vi "Compile 9759 RevB.vi"(8 "error in (no error)":errorcluster, 11 "Device Item Ref in":T2 format="%.0x") -> (0 "error out":errorcluster, 2 "9759 RevB":T1 {"Settings"."ControlCals"."ThetaLH (deg)" format="%.3f"; "Settings"."ControlCals"."ULHLag (sec)" format="%.3f"; "Settings"."ControlCals"."USLag (sec)" format="%.3f"; "Settings"."ControlCals"."TLead (sec)" format="%.3f"; "Settings"."ControlCals"."TLag (sec)" format="%.3f"}, 3 "Device Item Ref out":T2 format="%.0x")   [LabVIEW 2015, in "NI 9759 RevB Custom Device.lvlib"]
uses:
  NI 9759 RevB Custom Device.lvlib
  <vilib>/NI Veristand/Custom Device API/Custom Device Item Ref.ctl
  Shared/Types/9759 RevB.ctl
  Shared/9759 Constants and GUIDs.vi
  Shared/9759 Properties.vi
  <vilib>/NI VeriStand/Custom Device API/Custom Device API.lvlib
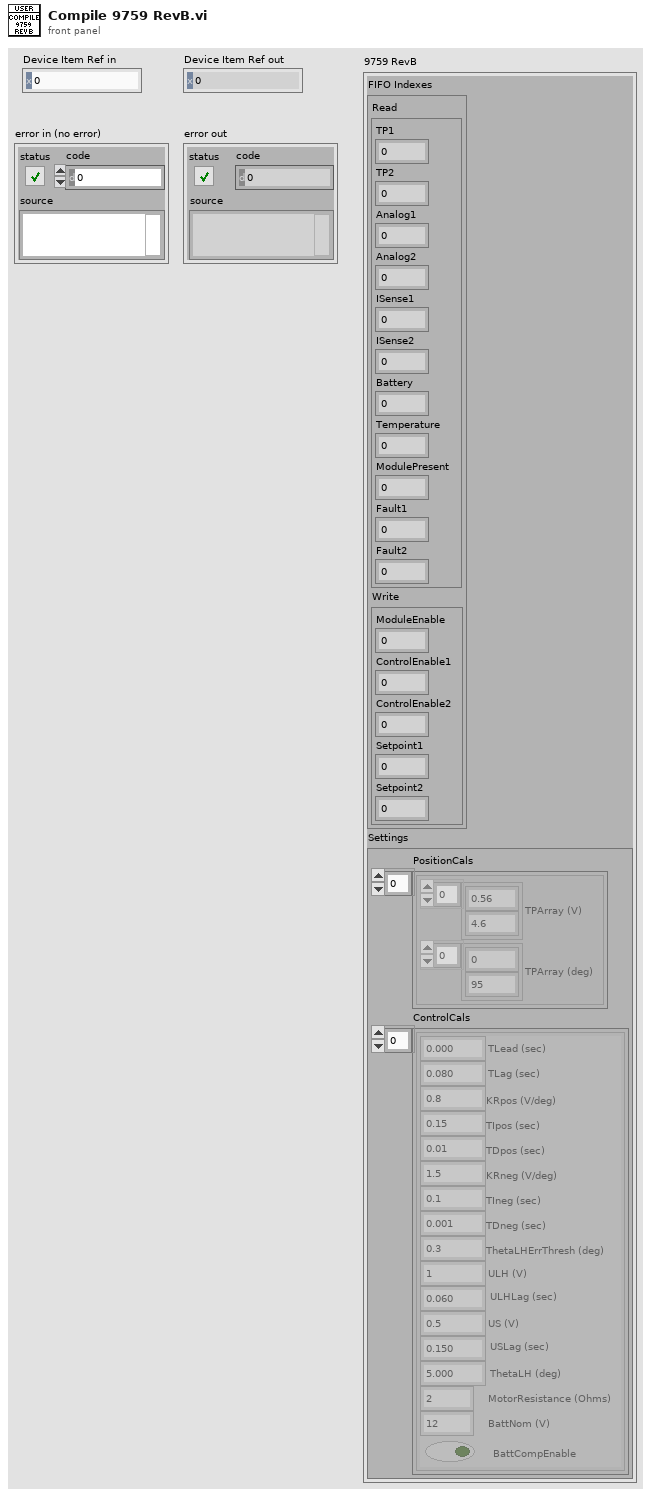
[diagram p1: front panel]
types:
  T1 = typedef "NI 9759 RevB Custom Device.lvlib/9759 RevB.ctl" = cluster{"FIFO Indexes":cluster{"Read":cluster{"TP1":i32, "TP2":i32, "Analog1":i32, "Analog2":i32, "ISense1":i32, "ISense2":i32, "Battery":i32, "Temperature":i32, "ModulePresent":i32, "Fault1":i32, "Fault2":i32}, "Write":cluster{"ModuleEnable":i32, "ControlEnable1":i32, "ControlEnable2":i32, "Setpoint1":i32, "Setpoint2":i32}}, "Settings":cluster{"PositionCals":cluster{"TPArray (V)":sgl[], "TPArray (deg)":sgl[]}[], "ControlCals":cluster{"TLead (sec)":sgl, "TLag (sec)":sgl, "KRpos (V/deg)":sgl, "TIpos (sec)":sgl, "TDpos (sec)":sgl, "KRneg (V/deg)":sgl, "TIneg (sec)":sgl, "TDneg (sec)":sgl, "ThetaLHErrThresh (deg)":sgl, "ULH (V)":sgl, "ULHLag (sec)":sgl, "US (V)":sgl, "USLag (sec)":sgl, "ThetaLH (deg)":sgl, "MotorResistance (Ohms)":sgl, "BattNom (V)":sgl, "BattCompEnable":bool}[]}}
  T2 = typedef "Custom Device API.lvlib/Custom Device Item Ref.ctl" = u64
  T3 = cluster{"TLead (sec)":sgl, "TLag (sec)":sgl, "KRpos (V/deg)":sgl, "TIpos (sec)":sgl, "TDpos (sec)":sgl, "KRneg (V/deg)":sgl, "TIneg (sec)":sgl, "TDneg (sec)":sgl, "ThetaLHErrThresh (deg)":sgl, "ULH (V)":sgl, "ULHLag (sec)":sgl, "US (V)":sgl, "USLag (sec)":sgl, "ThetaLH (deg)":sgl, "MotorResistance (Ohms)":sgl, "BattNom (V)":sgl, "BattCompEnable":bool}[]
  T4 = cluster{"TPArray (V)":sgl[], "TPArray (deg)":sgl[]}[]
  T5 = typedef "NI 9759 RevB Custom Device.lvlib/Channel.ctl" = cluster{"Name":string, "Units":string, "Default":dbl, "Description":string}
  T6 = cluster{"FIFO indexes[0]":i32, "FIFO indexes[1]":i32, "FIFO indexes[2]":i32, "FIFO indexes[3]":i32, "FIFO indexes[4]":i32}
  T7 = cluster{"FIFO indexes[0]":i32, "FIFO indexes[1]":i32, "FIFO indexes[2]":i32, "FIFO indexes[3]":i32, "FIFO indexes[4]":i32, "FIFO indexes[5]":i32, "FIFO indexes[6]":i32, "FIFO indexes[7]":i32, "FIFO indexes[8]":i32, "FIFO indexes[9]":i32, "FIFO indexes[10]":i32}
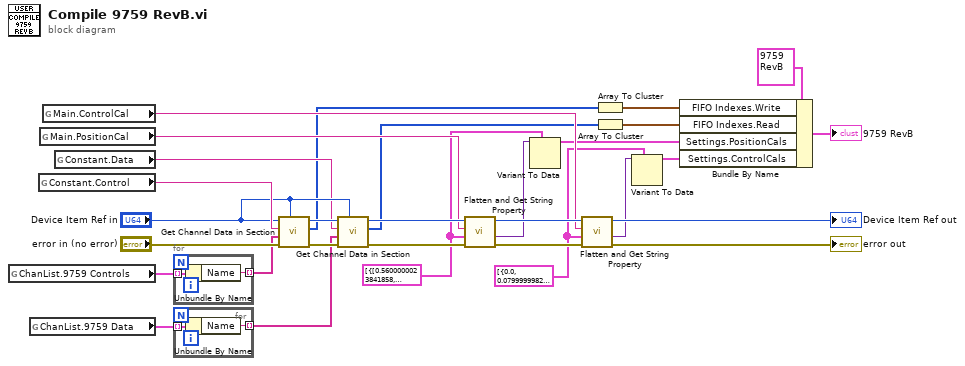
[diagram p0: block diagram]
diagram:
  w6 = T3 [{"TLead (sec)"=0.0, "TLag (sec)"=0.08, "KRpos (V/deg)"=0.8, "TIpos (sec)"=0.15, "TDpos (sec)"=0.01, "KRneg (V/deg)"=1.5, "TIneg (sec)"=0.1, "TDneg (sec)"=0.001, "ThetaLHErrThresh (deg)"=0.3, "ULH (V)"=1.0, "ULHLag (sec)"=0.06, "US (V)"=0.5, "USLag (sec)"=0.15, "ThetaLH (deg)"=5.0, "MotorResistance (Ohms)"=2.0, "BattNom (V)"=12.0, "BattCompEnable"=FALSE}, {"TLead (sec)"=0.0, "TLag (sec)"=0.08, "KRpos (V/deg)"=0.8, "TIpos (sec)"=0.15, "TDpos (sec)"=0.01, "KRneg (V/deg)"=1.5, "TIneg (sec)"=0.1, "TDneg (sec)"=0.001, "ThetaLHErrThresh (deg)"=0.3, "ULH (V)"=1.0, "ULHLag (sec)"=0.06, "US (V)"=0.5, "USLag (sec)"=0.15, "ThetaLH (deg)"=5.0, "MotorResistance (Ohms)"=2.0, "BattNom (V)"=12.0, "BattCompEnable"=FALSE}]
  w5 = T4 [{"TPArray (V)"=[0.56, 4.6], "TPArray (deg)"=[0.0, 95.0]}, {"TPArray (V)"=[0.56, 4.6], "TPArray (deg)"=[0.0, 95.0]}]
  n1 = global read "9759 Constants and GUIDs.vi" "ChanList.9759 Controls"() -> (w27:T5[])
  n2 = global read "9759 Constants and GUIDs.vi" "ChanList.9759 Data"() -> (w16:T5[])
  n3 = global read "9759 Constants and GUIDs.vi" "Constant.Control"() -> (w28:string)
  n4 = global read "9759 Properties.vi" "Main.PositionCal"() -> (w12:string)
  n5 = global read "9759 Properties.vi" "Main.ControlCal"() -> (w11:string)
  n6 = global read "9759 Constants and GUIDs.vi" "Constant.Data"() -> (w13:string)
  n7 = for {
    tunnel: w27 -> [w32] mode=indexing
    tunnel: [w31] -> w29 mode=indexing
    n8 = Unbundle By Name(w32) -> ("Name"=w31:string)
  }
  n9 = for {
    tunnel: w16 -> [w34] mode=indexing
    tunnel: [w33] -> w15 mode=indexing
    n10 = Unbundle By Name(w34) -> ("Name"=w33:string)
  }
  n11 = call "Get Channel Data in Section.vi"("Custom device ref"="Device Item Ref in", "error in (no error)"="error in (no error)", "Channels"=w29, "Section (\"\":none)"=w28, "Item Ref in"="Device Item Ref in") -> ("error out"=w17:errorcluster, "FIFO indexes"=w4:i32[], "Item Ref out"=w20:T2)  [unwired: 2 in, 2 out]
  n12 = call "Get Channel Data in Section.vi"("Custom device ref"="Device Item Ref in", "error in (no error)"=w17, "Channels"=w15, "Section (\"\":none)"=w13, "Item Ref in"=w20) -> ("error out"=w18:errorcluster, "FIFO indexes"=w3:i32[], "Item Ref out"=w19:T2)  [unwired: 2 in, 2 out]
  n13 = call "Flatten and Get String Property.vi"("error in (no error)"=w18, "Default Value"=w5, "Property Name"=w12, "Section Ref in"=w19) -> ("error out"=w22:errorcluster, "Value"=w8:variant, "Section Ref out"=w24:T2)  [unwired: 5 in]
  n14 = Variant To Data(type=w5, Variant=w8) -> (data=w10:T4)  [unwired: 1 in, 1 out]
  n15 = call "Flatten and Get String Property.vi"("error in (no error)"=w22, "Default Value"=w6, "Property Name"=w11, "Section Ref in"=w24) -> ("error out"=→"error out":errorcluster, "Value"=w9:variant, "Section Ref out"=→"Device Item Ref out":T2)  [unwired: 5 in]
  n16 = Array To Cluster(array=w4) -> (cluster=w1:T6)
  n17 = Array To Cluster(array=w3) -> (cluster=w2:T7)
  n18 = Variant To Data(type=w6, Variant=w9) -> (data=w7:T3)  [unwired: 1 in, 1 out]
  n19 = Bundle By Name(cluster=T1 {"FIFO Indexes"={"Read"={"TP1"=0, "TP2"=0, "Analog1"=0, "Analog2"=0, "ISense1"=0, "ISense2"=0, "Battery"=0, "Temperature"=0, "ModulePresent"=0, "Fault1"=0, "Fault2"=0}, "Write"={"ModuleEnable"=0, "ControlEnable1"=0, "ControlEnable2"=0, "Setpoint1"=0, "Setpoint2"=0}}, "Settings"={"PositionCals"=[], "ControlCals"=[]}} ("9759 RevB"), "FIFO Indexes.Write"=w1, "FIFO Indexes.Read"=w2, "Settings.PositionCals"=w10, "Settings.ControlCals"=w7) -> (→"9759 RevB":T1)
